vi "Force channel.vi"(6 "Degree":i16(ring) items=["0", "45", "90", "135", "180"], 7 "Vx":dbl, 8 "width/2":dbl=0.005, 9 "Y Value":dbl(slide) min=-5.0 max=5.0 step=1e-05 scale=0.0..5.0 scale format="%#.3g", 10 "X Value":dbl(slide) min=-5.0 max=5.0 step=1e-05 scale=0.0..5.0 scale format="%#.3g", 11 "Vy":dbl) -> (0 "Fy":dbl, 1 "Fx":dbl, 3 "In-range":bool)   [LabVIEW 2012]
uses:
  <vilib>/Analysis/coordinate.llb/2D Cartesian Coordinate Rotation (Scalar).vi
  <vilib>/Analysis/NI_AALPro.lvlib
  <userlib>/dhd323-32bit/dhd323-32bit.lvlib
panel:
  out "output-k":dbl
  in  "stiffness":dbl=2500.0
  in  "Type":i16 max=90 step=15
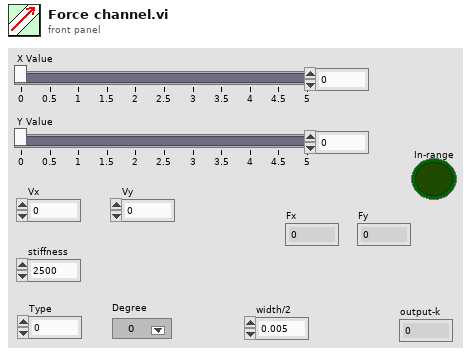
[diagram p1: front panel]
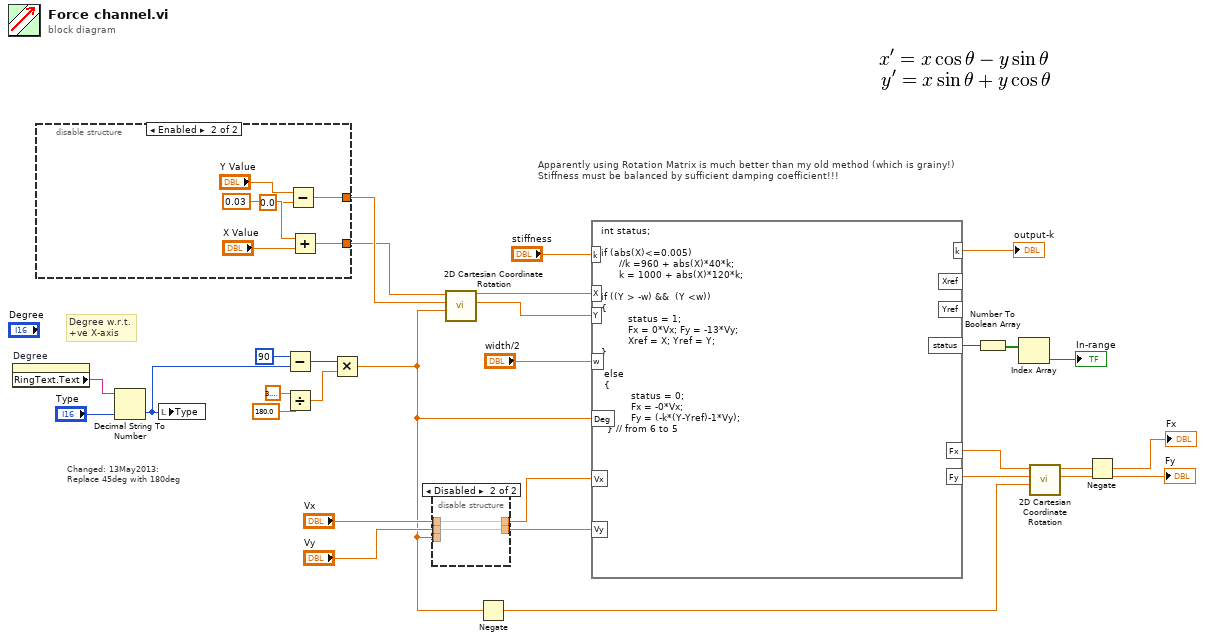
[diagram p0: block diagram]
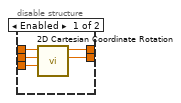
[diagram p2: hidden frame]
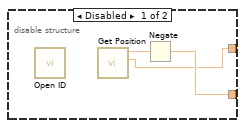
[diagram p3: hidden frame]
diagram:
  # "Changed: 13May2013:\nReplace 45deg with 180deg"
  # "Apparently using Rotation Matrix is much better than my old method (which is grainy!)\nStiffness must be balanced by sufficient damping coefficient!!!"
  # "Degree w.r.t.\n+ve X-axis"
  n1 = property on="Degree" class="Ring (strict)"() -> ("RingText.Text"=w29:string)  [unwired: 2 in, 2 out]
  n2 = disable-structure shown="Enabled" {
    disable-tunnel: [w30 w36] -> w27
    disable-tunnel: [w31 w35] -> w26
    frame Disabled {
      n3 = call <userlib>:"Open ID.vi"() -> ()  [unwired: 11 in, 1 out]
      n4 = call <userlib>:"Get Position.vi"() -> ("py out"=w30:dbl, "px out"=w32:dbl)  [unwired: 8 in, 2 out]
      n5 = Negate(x=w32) -> (-x=w31:dbl)
    }
    frame Enabled {
      n6 = Subtract(x="Y Value", y=0.0) -> (x-y=w36:dbl)
      n7 = Add(x=0.03 ("y"), y="X Value") -> (x+y=w35:dbl)
    }
  }
  n8 = Decimal String To Number(string=w29, default (0L)="Type") -> (number=w3:i16)  [unwired: 1 in, 1 out]
  n9 = local write "Type"(w3) -> ()
  n10 = Subtract(x=i16 90, y=w3) -> (x-y=w22:i16)
  n11 = Divide(x=3.141592653589793, y=180.0) -> (x/y=w23:dbl)
  n12 = Multiply(x=w22, y=w23) -> (x*y=w11:dbl)
  n13 = disable-structure shown="Disabled" {
    disable-tunnel: "Vx" -> [w43 w45]
    disable-tunnel: "Vy" -> [w42 w44]
    disable-tunnel: w11 -> [w41 _]
    disable-tunnel: [w40 w44] -> w10
    disable-tunnel: [w39 w45] -> w9
    frame Enabled {
      n14 = call-poly <vilib>:"2D Cartesian Coordinate Rotation.vi"("theta"=w41, "y"=w42, "x"=w43) -> ("y out"=w40:dbl, "x out"=w39:dbl)  [unwired: 6 in, 1 out]
    }
    frame Disabled {
    }
  }
  n15 = call-poly <vilib>:"2D Cartesian Coordinate Rotation.vi"("theta"=w11, "y"=w27, "x"=w26) -> ("y out"=w20:dbl, "x out"=w15:dbl)  [unwired: 6 in, 1 out]
  n16 = Negate(x=w11) -> (-x=w19:dbl)
  n17 = formula code="int status;\n \nif (abs(X)<=0.005)\n      //k =960 + abs(X)*40*k;\n      k = 1000 + abs(X)*120*k;\n\nif ((Y > -w) &&  (Y <w))\n{\n         status = 1;\n         Fx = 0*Vx; Fy = -13*Vy;\n         Xref = X; Yref = Y;\n}\n\n else \n { \n          status = 0;\n          Fx = -0*Vx;\n          Fy = (-k*(Y-Yref)-1*Vy);\n  } // from 6 to 5"("X"=w15, "Y"=w20, "Deg"=w11, "Vx"=w9, "Vy"=w10, "w"="width/2", "k"="stiffness") -> ("Fx"=w7:dbl, "Fy"=w8:dbl, "status"=w16:i32, "k"=→"output-k":dbl)  [unwired: 2 out]
  n18 = Number To Boolean Array(number=w16) -> (Boolean array=w17:bool[])
  n19 = Index Array(array=w17) -> (element=→"In-range":bool)  [unwired: 1 in]
  n20 = call-poly <vilib>:"2D Cartesian Coordinate Rotation.vi"("theta"=w19, "y"=w8, "x"=w7) -> ("y out"=→"Fy":dbl, "x out"=w6:dbl)  [unwired: 6 in, 1 out]
  n21 = Negate(x=w6) -> (-x=→"Fx":dbl)
